vi "control_indicator.vi"() -> ()   [LabVIEW 2019]
panel:
  out "String 2":string
  in  "String":string
  out "Boolean 2":bool
  in  "Boolean":bool
  out "a+b":dbl
  in  "b":dbl
  in  "a":dbl
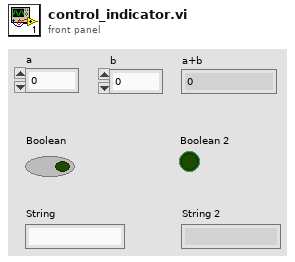
[diagram p1: front panel]
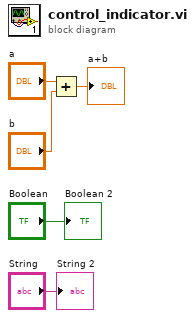
[diagram p0: block diagram]
diagram:
  n1 = Add(x="a", y="b") -> (x+y=→"a+b":dbl)
  "Boolean 2" <- "Boolean"
  "String 2" <- "String"
